vi "SIM921_Resistance_Bridge.vi"() -> ()   [LabVIEW 2019]
uses:
  Utility/Monitor Communication/SIM921/SIM921_resistance_Bridge_cluster.ctl
  Global/Global Variables/Data_Display_global.vi
  Instrument_Setup.vi
  Equipment/stanford_research_sim900_series/Stanford Research SIM900 Series/Stanford Research SIM900 Series.lvlib
panel:
  in  "stop":bool
  out "error out":errorcluster
  in  "error in (no error)":errorcluster
  in  "SIM921":T1
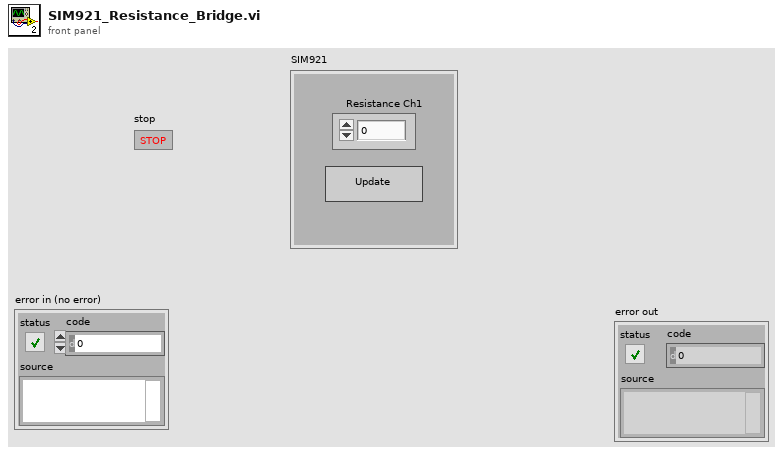
[diagram p1: front panel]
types:
  T1 = typedef "SIM921_resistance_Bridge_cluster.ctl" = cluster{"Resistance Ch1":dbl, "Update":bool}
  T2 = cluster{"SIM921-Address":refnum<visa-resource-name>, "SIM921-Channel 1 Port":dbl}
  T3 = typedef "SIM921_control_cluster.ctl" = cluster{"Update":bool}
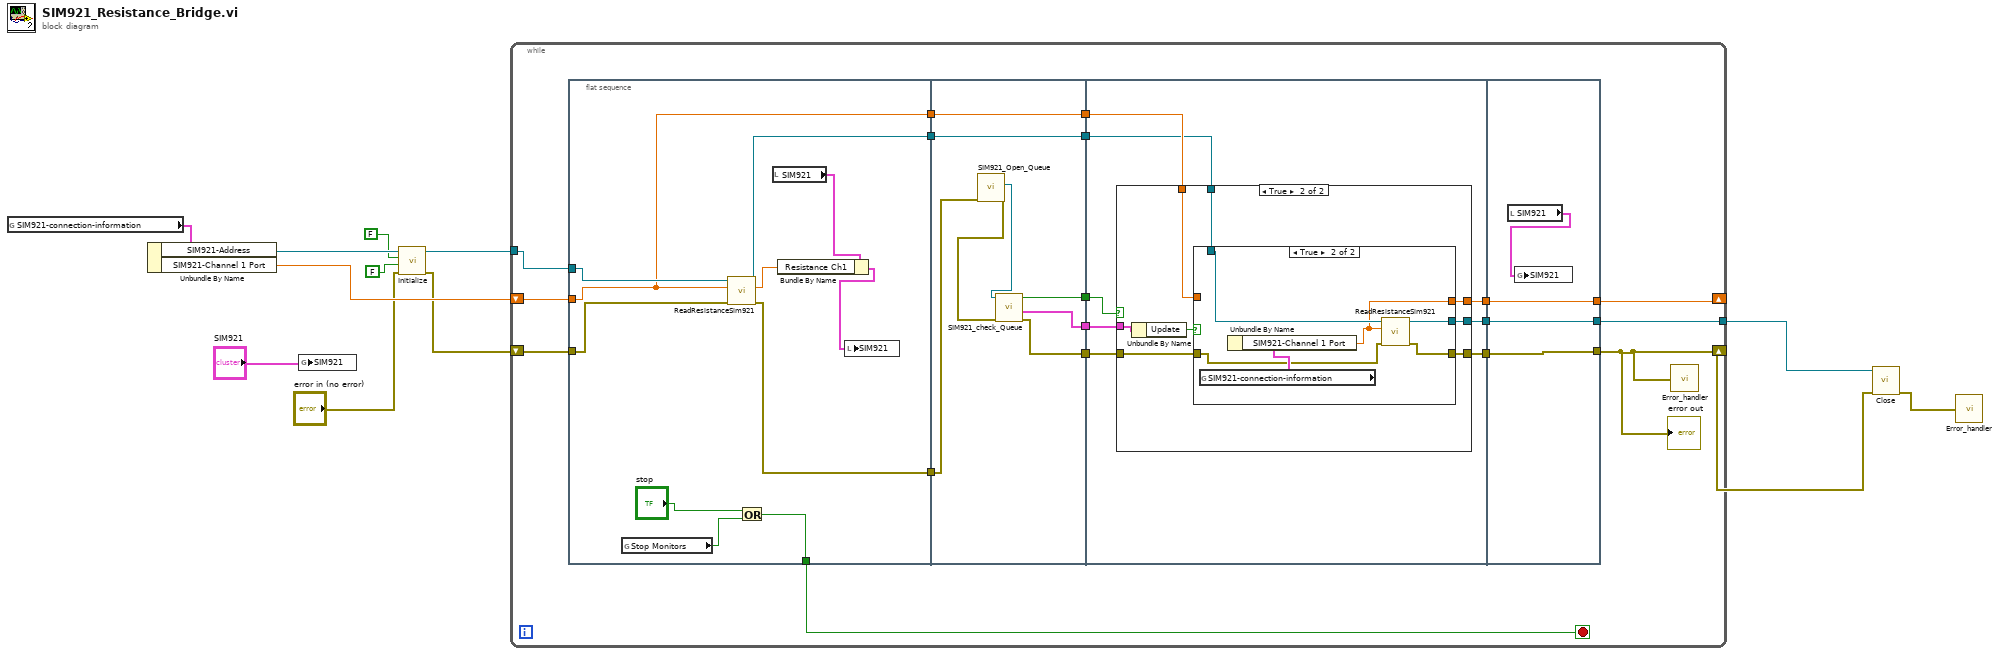
[diagram p0: block diagram]
diagram:
  n1 = global read "Instrument_Setup.vi" "SIM921-connection-information"() -> (w12:T2)
  n2 = Unbundle By Name(w12) -> ("SIM921-Address"=w11:refnum<visa-resource-name>, "SIM921-Channel 1 Port"=w9:dbl)
  n3 = global write "Data_Display_global.vi" "SIM921"("SIM921") -> ()
  n4 = call "Initialize.vi"("error in (no error)"="error in (no error)", "Reset (True)"=FALSE, "ID Query (True)"=FALSE, "VISA resource name"=w11) -> ("error out"=w1:errorcluster, "VISA resource name out"=w10:refnum<visa-resource-name>)  [unwired: 6 in]
  n5 = while {
    tunnel: w10 -> [w20]
    shift-right: [w23] -> w7
    shift-left: w1 -> [w29]
    shift-right: [w19] -> _
    shift-left: w9 -> [w30]
    tunnel: [w17] -> w6
    stop <- w18 stop-if-true
    n6 = flat-sequence {
      tunnel: w20 -> [w41]
      tunnel: w30 -> [w34]
      tunnel: w29 -> [w40]
      tunnel: [w39] -> w28
      tunnel: [w35] -> w27
      tunnel: [w34] -> w22
      tunnel: [w31] -> w18
      tunnel: w28 -> [w49]
      tunnel: w27 -> [w42]
      tunnel: [w46] -> w26
      tunnel: [w45] -> w25
      tunnel: [w44] -> w24
      tunnel: w22 -> [w43]
      tunnel: [w43] -> w21
      tunnel: [w42] -> w16
      tunnel: w26 -> [w57]
      tunnel: w25 -> [w54]
      tunnel: w24 -> [w56]
      tunnel: w21 -> [w53]
      tunnel: w16 -> [w50]
      tunnel: [w55] -> w15
      tunnel: [w52] -> w14
      tunnel: [w51] -> w13
      tunnel: [w79] -> w17
      tunnel: [w80] -> w19
      tunnel: [w81] -> w23
      tunnel: w15 -> [w81]
      tunnel: w14 -> [w80]
      tunnel: w13 -> [w79]
      frame #0 {
        n7 = global read "Data_Display_global.vi" "Stop Monitors"() -> (w32:bool)
        n8 = call "ReadResistanceSim921.vi"("error in (no error)"=w40, "Port"=w34, "GPIB"=w41) -> ("error out"=w39:errorcluster, "Resistance"=w36:dbl, "GPIB"=w35:refnum<visa-resource-name>)  [unwired: 5 in]
        n9 = Or(x="stop", y=w32) -> (x .or. y?=w31:bool)
        n10 = local read "SIM921"() -> (w38:T1)
        n11 = Bundle By Name(cluster=w38, "Resistance Ch1"=w36) -> (w37:T1)
        n12 = local write "SIM921"(w37) -> ()
      }
      frame #1 {
        n13 = call "SIM921_Open_Queue.vi"("error in (no error)"=w49) -> ("error out"=w48:errorcluster, "queue out"=w47:refnum<queue>)  [unwired: 9 in]
        n14 = call "SIM921_check_Queue.vi"("error in (no error)"=w48, "queue"=w47) -> ("error out"=w44:errorcluster, "SIM921-Control"=w45:T3, "New Entries ?"=w46:bool)  [unwired: 7 in]
      }
      frame #2 {
        n15 = case shown="True" w57 {
          tunnel: [w60 w65] -> w55
          tunnel: w56 -> [w60 w64]
          tunnel: w54 -> [_ w68]
          tunnel: w53 -> [w59 w66]
          tunnel: w50 -> [w58 w63]
          tunnel: [w59 w62] -> w52
          tunnel: [w58 w61] -> w51
          frame False {
          }
          frame True {
            n16 = Unbundle By Name(w68) -> ("Update"=w67:bool)
            n17 = case shown="True" w67 {
              tunnel: w66 -> [w71 _]
              tunnel: [w69 w76] -> w65
              tunnel: w64 -> [w69 w75]
              tunnel: w63 -> [w70 w74]
              tunnel: [w71 w73] -> w62
              tunnel: [w70 w72] -> w61
              frame False {
              }
              frame True {
                n18 = global read "Instrument_Setup.vi" "SIM921-connection-information"() -> (w77:T2)
                n19 = Unbundle By Name(w77) -> ("SIM921-Channel 1 Port"=w73:dbl)
                n20 = call "ReadResistanceSim921.vi"("error in (no error)"=w75, "Port"=w73, "GPIB"=w74) -> ("error out"=w76:errorcluster, "GPIB"=w72:refnum<visa-resource-name>)  [unwired: 5 in, 1 out]
              }
            }
          }
        }
      }
      frame #3 {
        n21 = local read "SIM921"() -> (w78:T1)
        n22 = global write "Data_Display_global.vi" "SIM921"(w78) -> ()
      }
    }
    n23 = call "Error_handler.vi"("error constant"=w23) -> ()
    "error out" <- w23
  }
  n24 = call "Close.vi"("error in (no error)"=w7, "VISA resource name"=w6) -> ("error out"=w8:errorcluster)  [unwired: 9 in]
  n25 = call "Error_handler.vi"("error constant"=w8) -> ()
